vi "Configure Spectrum Emission Mask (Offset Sweep Trace).vi"(0 "VISA resource name":refnum<visa-resource-name>, 1 "SEM Detect Mode":i32[](array[ring]) items=["Pos and Neg Peaks", "Positive Peaks", "Negative Peaks", "Sampling", "RMS"], 5 "SEM Sweep Time Select":i32[](array[ring]) items=["Normal", "Fast"], 7 "SEM Sweep Time Mode":i32[](array[ring]) items=["Off", "On"], 9 "SEM Sweep Time":dbl[](array[numeric]) min=0.001 max=1000.0, 11 "error in (no error)":errorcluster, 12 "SEM Trace Point":i32[](array[ring]) items=["11"=11, "21"=21, "41"=41, "51"=51, "201"=201, "251"=251, "401"=401, "501"=501, "1001"=1001, "2001"=2001, "5001"=5001, "10001"=10001]) -> (4 "VISA resource name out":refnum<visa-resource-name>, 15 "error out":errorcluster)   [LabVIEW 2020, in "Anritsu Signal Analyzer Series.lvlib"]
doc: "Configures the setup for offset sweep trace of SEM measurement settings of the spectrum analyzer."
uses:
  Anritsu Signal Analyzer Series.lvlib
panel:
  # "s"
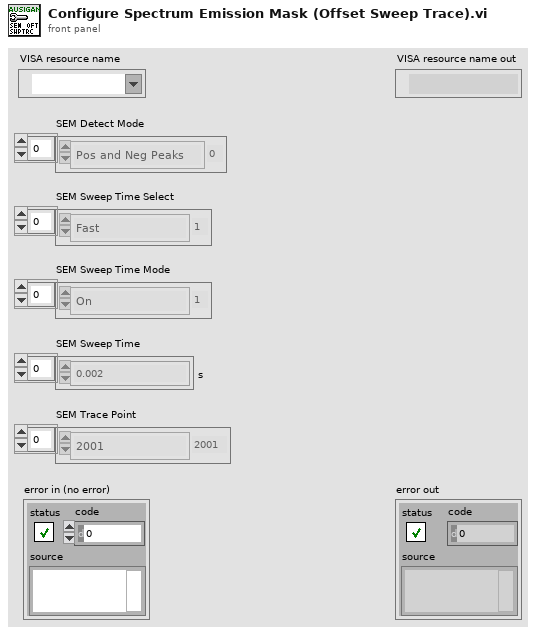
[diagram p1: front panel]
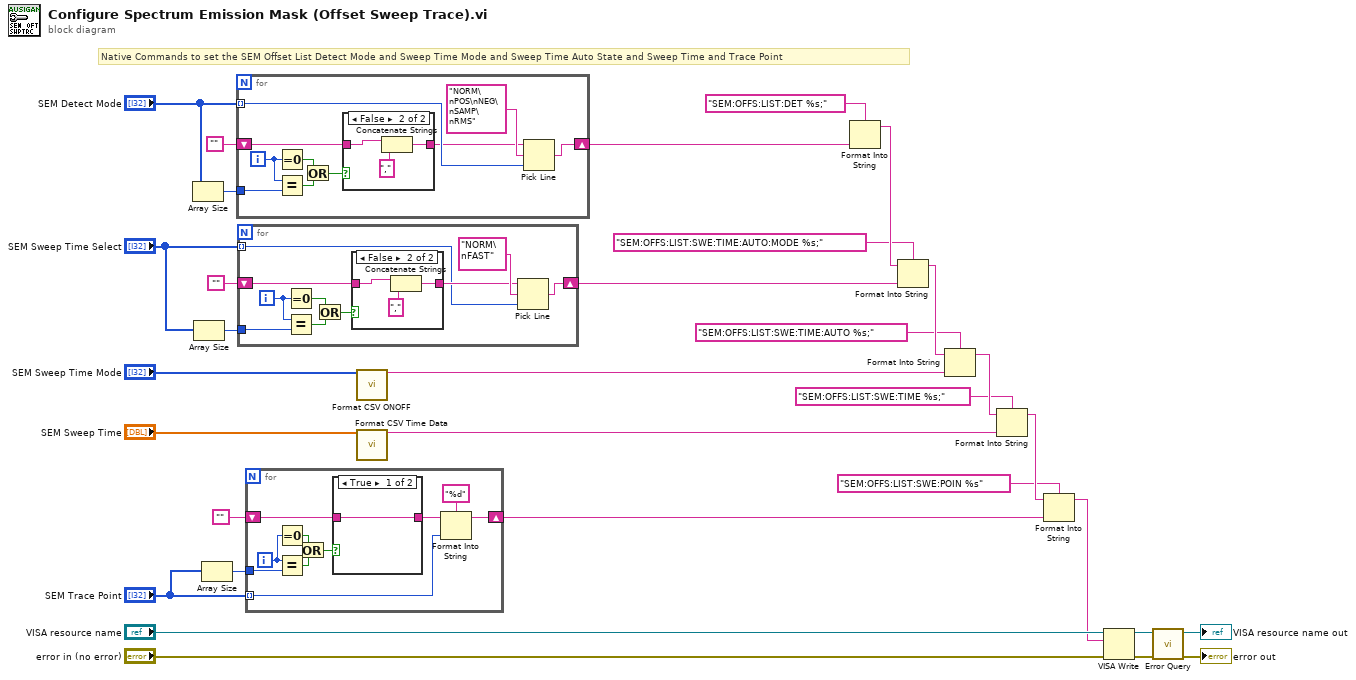
[diagram p0: block diagram]
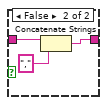
[diagram p2: hidden frame]
diagram:
  # "Native Commands to set the SEM Offset List Detect Mode and Sweep Time Mode and Sweep Time Auto State and Sweep Time and Trace Point"
  n1 = Array Size(array="SEM Detect Mode") -> (size(s)=w22:i32)
  n2 = Array Size(array="SEM Sweep Time Select") -> (size(s)=w9:i32)
  n3 = Array Size(array="SEM Trace Point") -> (size(s)=w4:i32)
  n4 = for {
    tunnel: "SEM Detect Mode" -> [w35] mode=indexing
    shift-right: [w33] -> w10
    shift-left: "" -> [w42]
    tunnel: w22 -> [w37]
    i -> [w38]
    n5 = Equal To 0?(x=w38) -> (x = 0?=w41:bool)
    n6 = Equal?(x=w38, y=w37) -> (x = y?=w40:bool)
    n7 = Or(x=w41, y=w40) -> (x .or. y?=w39:bool)
    n8 = case shown="False" w39 {
      tunnel: w42 -> [w43 w46]
      tunnel: [w43 w44] -> w34
      frame True {
      }
      frame False {
        n9 = Concatenate Strings(w46, "," ("string")) -> (w44:string)
      }
    }
    n10 = Pick Line(string ("")=w34, multi-line string="NORM\nPOS\nNEG\nSAMP\nRMS" ("複数行文字列"), line index=w35) -> (output string=w33:string)
  }
  n11 = for {
    tunnel: "SEM Sweep Time Select" -> [w47] mode=indexing
    shift-right: [w48] -> w7
    shift-left: "" -> [w56]
    tunnel: w9 -> [w51]
    i -> [w52]
    n12 = Equal To 0?(x=w52) -> (x = 0?=w55:bool)
    n13 = Equal?(x=w52, y=w51) -> (x = y?=w54:bool)
    n14 = Or(x=w55, y=w54) -> (x .or. y?=w53:bool)
    n15 = case shown="False" w53 {
      tunnel: w56 -> [w57 w60]
      tunnel: [w57 w58] -> w49
      frame True {
      }
      frame False {
        n16 = Concatenate Strings(w60, "," ("string")) -> (w58:string)
      }
    }
    n17 = Pick Line(string ("")=w49, multi-line string="NORM\nFAST" ("複数行文字列"), line index=w47) -> (output string=w48:string)
  }
  n18 = for {
    shift-right: [w67] -> w3
    shift-left: "" -> [w70]
    tunnel: w4 -> [w66]
    tunnel: "SEM Trace Point" -> [w61] mode=indexing
    i -> [w62]
    n19 = Equal To 0?(x=w62) -> (x = 0?=w65:bool)
    n20 = Equal?(x=w62, y=w66) -> (x = y?=w64:bool)
    n21 = Or(x=w65, y=w64) -> (x .or. y?=w63:bool)
    n22 = case shown="True" w63 {
      tunnel: w70 -> [w71 w74]
      tunnel: [w71 w72] -> w69
      frame True {
      }
      frame False {
        n23 = Concatenate Strings(w74, "," ("string")) -> (w72:string)
      }
    }
    n24 = Format Into String(format string="%d", initial string=w69, w61) -> (resulting string=w67:string)  [unwired: 1 in, 1 out]
  }
  n25 = call "Format CSV ONOFF.vi"("Data_In"="SEM Sweep Time Mode") -> ("Data_out"=w11:string)  [unwired: 14 in]
  n26 = call "Format CSV Time Data.vi"("Data_In"="SEM Sweep Time") -> ("Data_out"=w6:string)  [unwired: 14 in]
  n27 = Format Into String(format string="SEM:OFFS:LIST:DET %s;" ("_CommandSet"), w10) -> (resulting string=w20:string)  [unwired: 2 in, 1 out]
  n28 = Format Into String(format string="SEM:OFFS:LIST:SWE:TIME:AUTO:MODE %s;" ("_CommandSet"), initial string=w20, w7) -> (resulting string=w18:string)  [unwired: 1 in, 1 out]
  n29 = Format Into String(format string="SEM:OFFS:LIST:SWE:TIME:AUTO %s;" ("_CommandSet"), initial string=w18, w11) -> (resulting string=w16:string)  [unwired: 1 in, 1 out]
  n30 = Format Into String(format string="SEM:OFFS:LIST:SWE:TIME %s;" ("_CommandSet"), initial string=w16, w6) -> (resulting string=w14:string)  [unwired: 1 in, 1 out]
  n31 = Format Into String(format string="SEM:OFFS:LIST:SWE:POIN %s" ("_CommandSet"), initial string=w14, w3) -> (resulting string=w12:string)  [unwired: 1 in, 1 out]
  n32 = VISA Write(VISA resource name="VISA resource name", write buffer=w12, error in (no error)="error in (no error)") -> (VISA resource name out=w2:refnum<visa-resource-name>, error out=w1:errorcluster)  [unwired: 1 out]
  n33 = call "Error Query.vi"("error in (no error)"=w1, "VISA resource name"=w2) -> ("error out"=→"error out":errorcluster, "VISA resource name out"=→"VISA resource name out":refnum<visa-resource-name>)  [unwired: 6 in, 2 out]
